vi "Teleop.vi"(10 "Match Info":T1={"Autonomous Elapsed Seconds"=0.0, "TeleOp Elapsed Seconds"=0.0, "Disabled Elapsed Seconds"=0.0, "Visited Autonomous"=FALSE, "Visited TeleOp"=FALSE, "Visited Disabled"=FALSE, "Autonomous Settings"={"Autonomous Style"=enum."Independent", "VI Refnum"=refnum}}, 11 "Call Context":T2) -> ()   [LabVIEW 2017]
doc: "This VI is called for each TeleOp packet received from the DS where the robot is not disabled. It is often used to read from the joysticks and update I/O or to update setpoints for timed control loops. It should complete and return within 20 milliseconds or it may miss DS packets."
uses:
  <vilib>/Rock Robotics/WPI/DriverStation/WPI_DriverStationDerivedRobotMode.ctl
  <vilib>/Rock Robotics/WPI/DriverStation/WPI_DriverStationMatch Info.ctl
  Phoenix-LabVIEW/Motor Controller/Controls/CTRE_Phoenix_MotorControl_ControlMode.ctl
  <vilib>/Rock Robotics/WPI/ThirdParty/Sensors/navX/_TypeDefs/FRIC_navX_DeviceNumbersTypeDef.ctl
  <vilib>/Rock Robotics/WPI/Utilities/WPI_GetSetVariantRefNum.vi
panel:
  in  "LiftSpeed":dbl=1.0 format="%#_13g"
  in  "LiftSetpoint":dbl=0.45 format="%#_13g"
  in  "Lift PID":bool
  in  "WristSetpoint":dbl format="%#_13g"
  in  "WristSpeed":dbl=1.0 format="%#_13g"
  in  "Wrist PID":bool
  out "RightOut":dbl
  out "LeftOut":dbl
  in  "K Constant":dbl=-1.0 format="%#_13g"
  in  "Deadband":dbl=0.05 format="%#_13g"
  in  "DriveSpeed":dbl=0.95 format="%#_13g"
  in  "IntakeSpeed":dbl=0.9
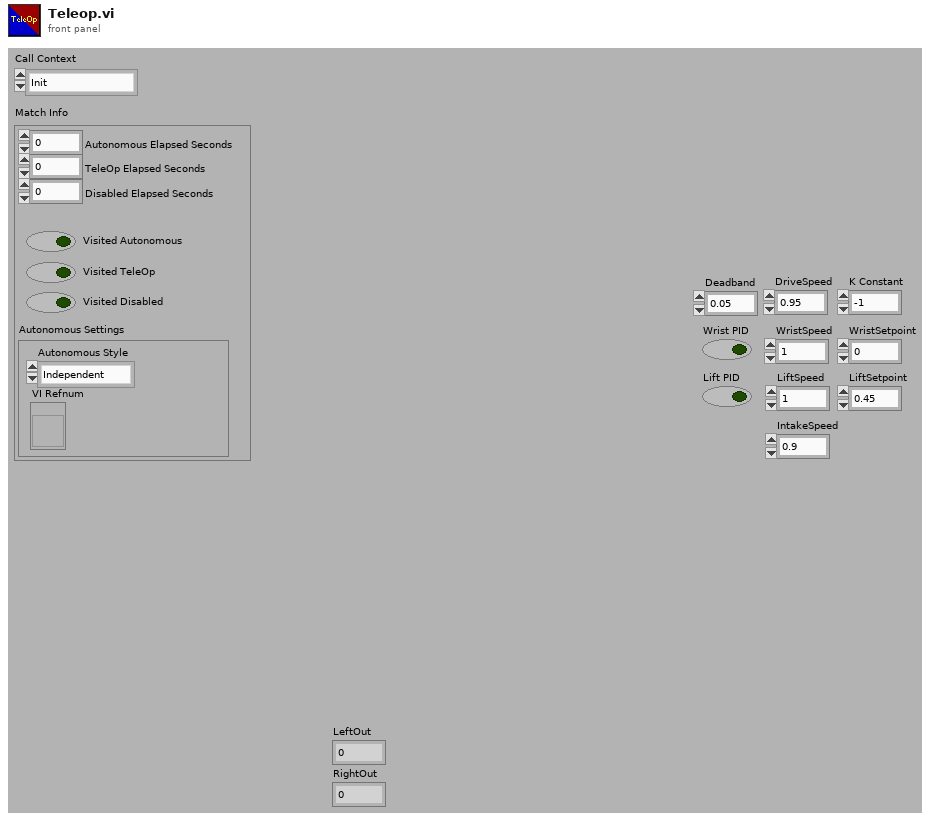
[diagram p1: front panel]
types:
  T1 = typedef "WPI_DriverStationMatch Info.ctl" = cluster{"Autonomous Elapsed Seconds":dbl, "TeleOp Elapsed Seconds":dbl, "Disabled Elapsed Seconds":dbl, "Visited Autonomous":bool, "Visited TeleOp":bool, "Visited Disabled":bool, "Autonomous Settings":cluster{"Autonomous Style":enum16{"Iterative", "Independent"}, "VI Refnum":refnum<vi>}}
  T2 = typedef "WPI_DriverStationDerivedRobotMode.ctl" = enum16{"Init", "Execute", "Stop"}
  T3 = typedef "CTRE_Phoenix_MotorControl_ControlMode.ctl" = u16
  T4 = typedef "WPI_JoystickDevRef.ctl" = cluster{"Device":T5}
  T5 = typedef "WPI_JoystickDeviceEnum.ctl" = enum16{"USB 0", "USB 1", "USB 2", "USB 3", "USB 4", "USB 5"}
  T6 = cluster{"Axes[0]":dbl, "Axes[1]":dbl, "Axes[2]":dbl, "Axes[3]":dbl, "Axes[4]":dbl, "Axes[5]":dbl, "Axes[6]":dbl, "Axes[7]":dbl, "Axes[8]":dbl}
  T7 = cluster{"Buttons[0]":bool, "Buttons[1]":bool, "Buttons[2]":bool, "Buttons[3]":bool, "Buttons[4]":bool, "Buttons[5]":bool, "Buttons[6]":bool, "Buttons[7]":bool, "Buttons[8]":bool}
  T8 = typedef "FRIC_navX_DeviceNumbersTypeDef.ctl" = enum16{"Dev0", "Dev1", "Dev2", "Dev3"}
  T9 = typedef "WPI_MotorControlDeviceRef.ctl" = cluster{"DeviceStatus":errorcluster, "Type":T10, "PWM":cluster{"PWM Channel":T11, "DeadBand":T12}, "CAN":cluster{"Device Number":u8, "SetOutput VI Ref":variant, "GetOutput VI Ref":variant, "Enable VI Ref":variant, "Disable VI Ref":variant, "Data":variant}, "Invert":bool, "DIO PWM":cluster{"PWM \"Enable\" Channel":T11, "DIOChannel":T13, "PWM Rate":dbl}}
  T10 = typedef "WPI_MotorControlType.ctl" = enum16{"PWM", "CAN", "DIO PWM"}
  T11 = typedef "FPGA_DIOPWMChannel.ctl" = enum8{"PWM 0", "PWM 1", "PWM 2", "PWM 3", "PWM 4", "PWM 5", "PWM 6", "PWM 7", "PWM 8", "PWM 9", "PWM MXP 0", "PWM MXP 1", "PWM MXP 2", "PWM MXP 3", "PWM MXP 4", "PWM MXP 5", "PWM MXP 6", "PWM MXP 7", "PWM MXP 8", "PWM MXP 9", "Invalid"}
  T12 = typedef "WPI_PWMDeadband.ctl" = cluster{"Name":string, "maxPositivePwm":i32, "minPositivePwm":i32, "centerPwm":i32, "maxNegativePwm":i32, "minNegativePwm":i32, "angularRange":u16}
  T13 = typedef "FPGA_DIOChannel.ctl" = enum8{"DIO 0", "DIO 1", "DIO 2", "DIO 3", "DIO 4", "DIO 5", "DIO 6", "DIO 7", "DIO 8", "DIO 9", "DIO MXP 0", "DIO MXP 1", "DIO MXP 2", "DIO MXP 3", "DIO MXP 4", "DIO MXP 5", "DIO MXP 6", "DIO MXP 7", "DIO MXP 8", "DIO MXP 9", "DIO MXP 10", "DIO MXP 11", "DIO MXP 12", "DIO MXP 13", "DIO MXP 14", "DIO MXP 15", "SPI Port CS1", "SPI Port CS2", "SPI Port CS3", "SPI Port MISO", "SPI Port MOSI", "Invalid"}
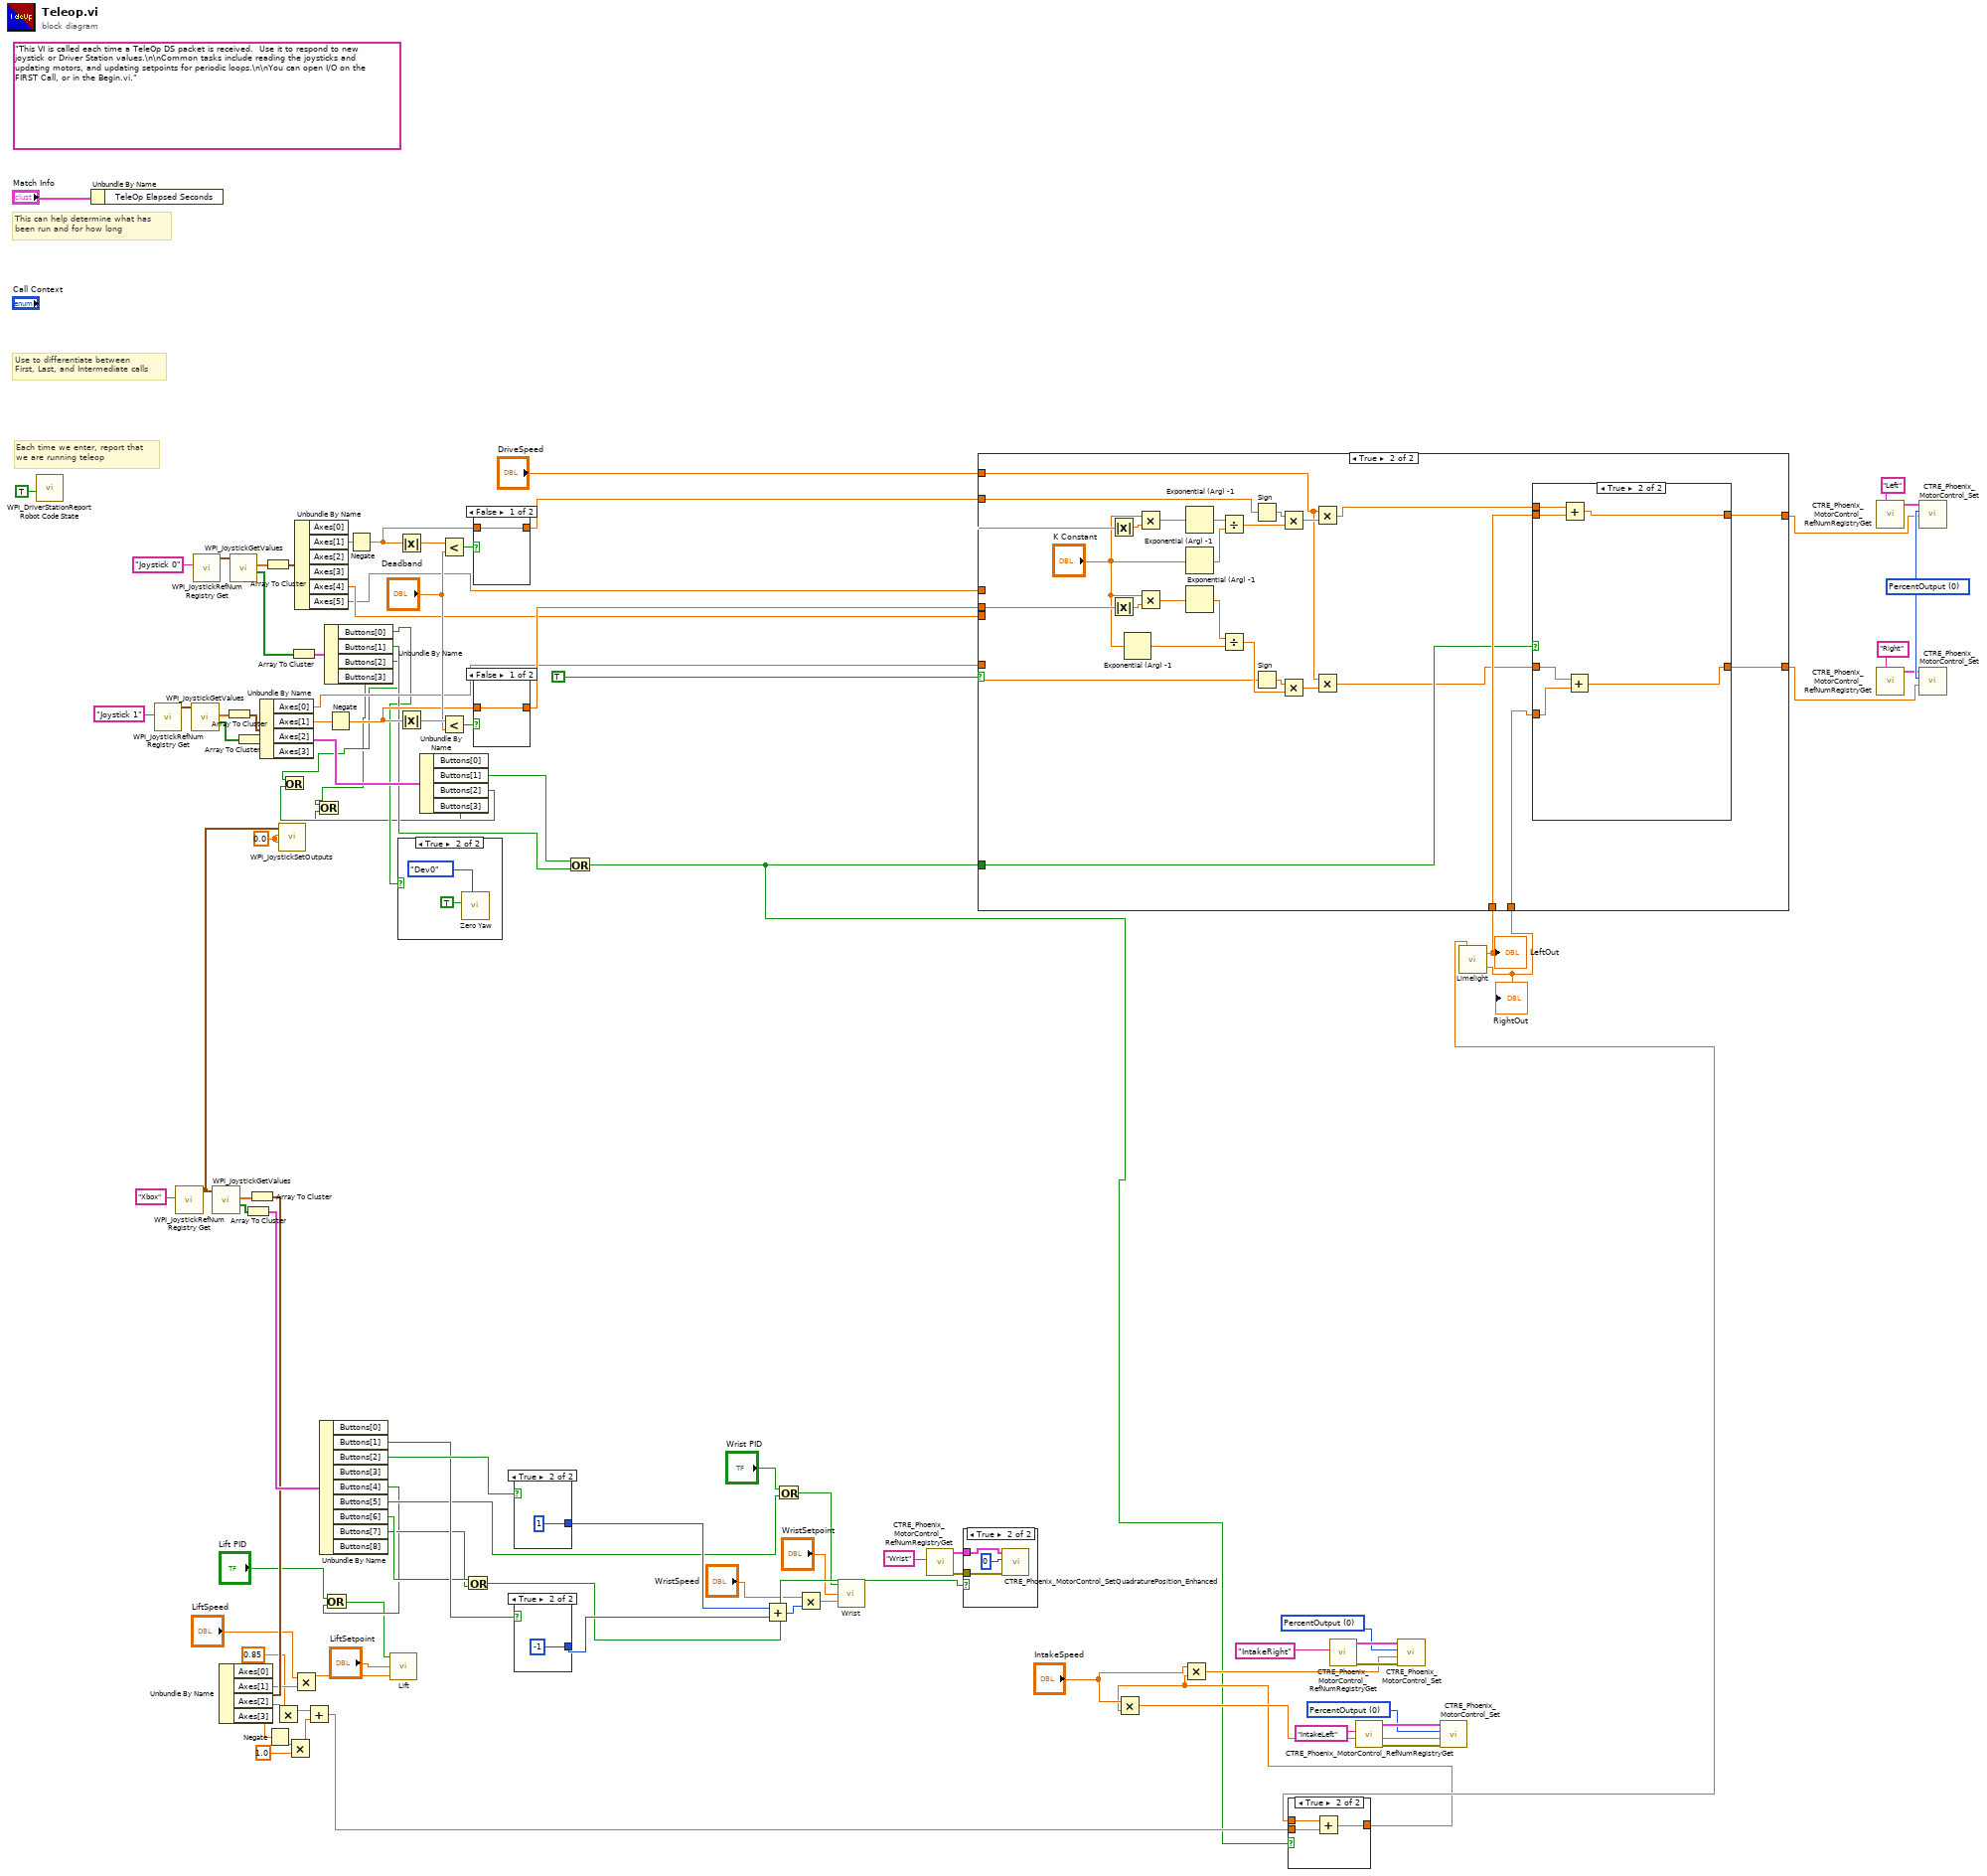
[diagram p0: block diagram]
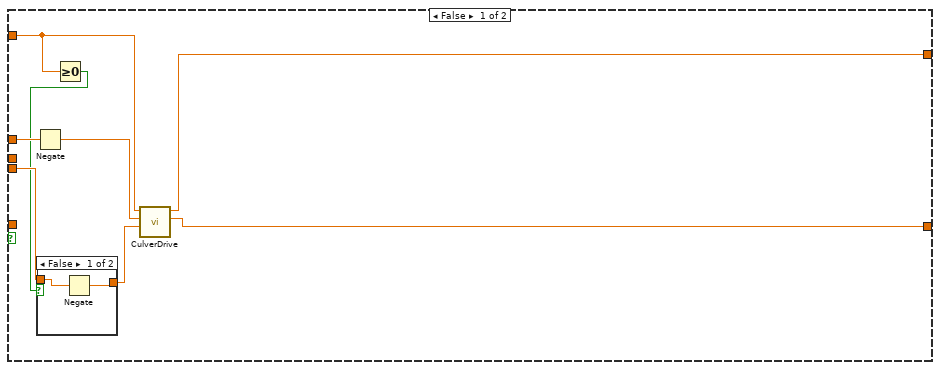
[diagram p5: hidden frame]
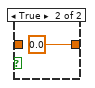
[diagram p8: hidden frame]
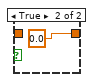
[diagram p9: hidden frame]
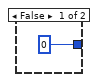
[diagram p10: hidden frame]
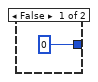
[diagram p11: hidden frame]
diagram:
  w48 = sgl 0.0 ("Left Rumble")
  w82 = T3 0 items=["PercentOutput"=0, "Position"=1, "Velocity"=2, "Current"=3, "Follower"=5, "MotionProfile"=6, "MotionMagic"=7, "MotionMagicArc"=8, "MotionProfileArc"=10, "Disabled"=15] ("Control Mode")
  w85 = T3 0 items=["PercentOutput"=0, "Position"=1, "Velocity"=2, "Current"=3, "Follower"=5, "MotionProfile"=6, "MotionMagic"=7, "MotionMagicArc"=8, "MotionProfileArc"=10, "Disabled"=15] ("Control Mode")
  w89 = T3 0 items=["PercentOutput"=0, "Position"=1, "Velocity"=2, "Current"=3, "Follower"=5, "MotionProfile"=6, "MotionMagic"=7, "MotionMagicArc"=8, "MotionProfileArc"=10, "Disabled"=15] ("Control Mode")
  (unwired) "This VI is called each time a TeleOp DS packet is received.  Use it to respond to new joystick or Driver Station values.\n\nCommon tasks include reading the joysticks and updating motors, and updating setpoints for periodic loops.\n\nYou can open I/O on the FIRST Call, or in the Begin.vi."
  # "Each time we enter, report that\nwe are running teleop"
  # "Use to differentiate between\nFirst, Last, and Intermediate calls"
  # "This can help determine what has\nbeen run and for how long"
  n1 = call <vilib>:"WPI_DriverStationReport Robot Code State.vi"("TeleOp"=TRUE ("Autonomous")) -> ()  [unwired: 10 in, 1 out]
  n2 = Unbundle By Name("Match Info") -> ()  [unwired: 1 out]
  n3 = call <vilib>:"WPI_JoystickRefNum Registry Get.vi"("refnum name"="Joystick 1") -> ("JoystickDevRef"=w52:T4)  [unwired: 1 in, 9 out]
  n4 = call <vilib>:"WPI_JoystickRefNum Registry Get.vi"("refnum name"="Xbox") -> ("JoystickDevRef"=w49:T4)  [unwired: 1 in, 9 out]
  n5 = call <vilib>:"WPI_JoystickGetValues.vi"("JoystickDevRef"=w52) -> ("Buttons"=w56:bool[], "Axes"=w76:dbl[])  [unwired: 6 in, 3 out]
  n6 = call <vilib>:"WPI_JoystickRefNum Registry Get.vi"("refnum name"="Joystick 0") -> ("JoystickDevRef"=w53:T4)  [unwired: 1 in, 9 out]
  n7 = call <vilib>:"WPI_JoystickGetValues.vi"("JoystickDevRef"=w49) -> ("Buttons"=w69:bool[], "Axes"=w70:dbl[])  [unwired: 6 in, 3 out]
  n8 = Array To Cluster(array=w76) -> (cluster=w75:T6)
  n9 = call <vilib>:"WPI_JoystickGetValues.vi"("JoystickDevRef"=w53) -> ("Buttons"=w80:bool[], "Axes"=w81:dbl[])  [unwired: 6 in, 3 out]
  n10 = Array To Cluster(array=w56) -> (cluster=w55:T7)
  n11 = Array To Cluster(array=w69) -> (cluster=w68:T7)
  n12 = Array To Cluster(array=w70) -> (cluster=w67:T6)
  n13 = Unbundle By Name(w67) -> ("Axes[1]"=w12:dbl, "Axes[2]"=w43:dbl, "Axes[3]"=w42:dbl)  [unwired: 1 out]
  n14 = Unbundle By Name(w75) -> ("Axes[0]"=w46:dbl, "Axes[1]"=w57:dbl)  [unwired: 2 out]
  n15 = Array To Cluster(array=w81) -> (cluster=w79:T6)
  n16 = Negate(x=w42) -> (-x=w4:dbl)
  n17 = Multiply(x=w43, y=0.85) -> (x*y=w2:dbl)
  n18 = call <vilib>:"WPI_JoystickSetOutputs.vi"("Right Rumble"=w48, "Left Rumble"=w48, "JoystickDevRef"=w49) -> ()  [unwired: 7 in, 2 out]
  n19 = Multiply(x=w4, y=1.0) -> (x*y=w5:dbl)
  n20 = Array To Cluster(array=w80) -> (cluster=w78:T7)
  n21 = Multiply(x="LiftSpeed", y=w12) -> (x*y=w7:dbl)
  n22 = Unbundle By Name(w79) -> ("Axes[1]"=w59:dbl, "Axes[4]"=w45:dbl, "Axes[5]"=w44:dbl)  [unwired: 3 out]
  n23 = Add(x=w2, y=w5) -> (x+y=w41:dbl)
  n24 = Unbundle By Name(w68) -> ("Buttons[1]"=w66:bool, "Buttons[2]"=w94:bool, "Buttons[4]"=w10:bool, "Buttons[5]"=w21:bool, "Buttons[6]"=w27:bool, "Buttons[7]"=w26:bool)  [unwired: 3 out]
  n25 = Or(x="Lift PID", y=w10) -> (x .or. y?=w9:bool)
  n26 = Unbundle By Name(w78) -> ("Buttons[0]"=w33:bool, "Buttons[1]"=w38:bool, "Buttons[2]"=w32:bool, "Buttons[3]"=w30:bool)
  n27 = Negate(x=w57) -> (-x=w50:dbl)
  n28 = Negate(x=w59) -> (-x=w51:dbl)
  n29 = call "Lift.vi"("LiftInput"=w7, "LiftSet"="LiftSetpoint", "LiftSweet"=w9) -> ()
  n30 = Absolute Value(x=w51) -> (abs(x)=w64:dbl)
  n31 = Absolute Value(x=w50) -> (abs(x)=w62:dbl)
  n32 = case shown="True" w33 {
    frame False {
    }
    frame True {
      n33 = call <vilib>:"Zero Yaw.vi"("Device Number"=FRIC_navX_DeviceNumbersTypeDef."Dev0", "Zero"=TRUE) -> ()  [unwired: 10 in]
    }
  }
  n34 = Unbundle By Name(w55) -> ("Buttons[1]"=w54:bool, "Buttons[2]"=w31:bool, "Buttons[3]"=w29:bool)  [unwired: 1 out]
  n35 = Or(x=w32, y=w31) -> ()  [unwired: 1 out]
  n36 = Or(x=w30, y=w29) -> ()  [unwired: 1 out]
  n37 = Less?(x=w64, y="Deadband") -> (x < y?=w65:bool)
  n38 = Less?(x=w62, y="Deadband") -> (x < y?=w63:bool)
  n39 = Or(x=w27, y=w26) -> (x .or. y?=w25:bool)
  n40 = case shown="False" w65 {
    tunnel: w51 -> [w102 _]
    tunnel: [w102 0.0] -> w61
    frame False {
    }
    frame True {
    }
  }
  n41 = case shown="False" w63 {
    tunnel: w50 -> [w104 _]
    tunnel: [w104 0.0] -> w60
    frame False {
    }
    frame True {
    }
  }
  n42 = case shown="True" w94 {
    tunnel: [0 1] -> w92
    frame False {
    }
    frame True {
    }
  }
  n43 = case shown="True" w66 {
    tunnel: [0 -1] -> w95
    frame False {
    }
    frame True {
    }
  }
  n44 = Or(x=w54, y=w38) -> (x .or. y?=w34:bool)
  n45 = Add(x=w92, y=w95) -> (x+y=w19:i32)
  n46 = Or(x="Wrist PID", y=w21) -> (x .or. y?=w20:bool)
  n47 = Multiply(x="WristSpeed", y=w19) -> (x*y=w18:dbl)
  n48 = call "Wrist.vi"("WristInput"=w18, "WristSetpoint"="WristSetpoint", "WristSweet"=w20) -> ()
  n49 = call "CTRE_Phoenix_MotorControl_RefNumRegistryGet.vi"("refnum name"="Wrist") -> ("error out"=w13:errorcluster, "PhoenixMotorControlDevRef"=w14:T9)  [unwired: 9 in]
  n50 = case shown="True" w25 {
    tunnel: w14 -> [_ w111]
    tunnel: w13 -> [_ w110]
    frame False {
    }
    frame True {
      n51 = call <vilib>:"CTRE_Phoenix_MotorControl_SetQuadraturePosition_Enhanced.vi"("error in (no error)"=w110, "New Position"=0, "PhoenixMotorControlDevRef"=w111) -> ()  [unwired: 7 in, 2 out]
    }
  }
  n52 = call "CTRE_Phoenix_MotorControl_RefNumRegistryGet.vi"("refnum name"="IntakeRight") -> ("error out"=w90:errorcluster, "PhoenixMotorControlDevRef"=w91:T9)  [unwired: 9 in]
  n53 = call "CTRE_Phoenix_MotorControl_RefNumRegistryGet.vi"("refnum name"="IntakeLeft") -> ("error out"=w86:errorcluster, "PhoenixMotorControlDevRef"=w87:T9)  [unwired: 9 in]
  n54 = call "Limelight.vi"() -> ("RightOut"=w39:dbl, "LeftOut"=w40:dbl, "IntakeOut"=w36:dbl)  [unwired: 1 in]
  "LeftOut" <- w40
  "RightOut" <- w39
  n55 = case shown="True" TRUE {
    tunnel: w61 -> [w116 w136]
    tunnel: w60 -> [_ w135]
    tunnel: [w119 w128] -> w23
    tunnel: [w120 w130] -> w24
    tunnel: w46 -> [_ _]
    tunnel: w45 -> [w115 _]
    tunnel: w44 -> [w118 _]
    tunnel: w40 -> [_ w131]
    tunnel: w39 -> [_ w129]
    tunnel: w34 -> [_ w127]
    tunnel: "DriveSpeed" -> [_ w124]
    frame False {
      n56 = Negate(x=w118) -> (-x=w117:dbl)
      n57 = Greater Or Equal To 0?(x=w116) -> (x >= 0?=w114:bool)
      n58 = case shown="False" w114 {
        tunnel: w115 -> [w121 w123]
        tunnel: [w122 w123] -> w113
        frame False {
          n59 = Negate(x=w121) -> (-x=w122:dbl)
        }
        frame True {
        }
      }
      n60 = call "CulverDrive.vi"("Wheel.X"=w113, "Wheel.Y"=w117, "Throttle"=w116) -> ("Right Side"=w119:dbl, "Left Side"=w120:dbl)  [unwired: 5 in, 2 out]
    }
    frame True {
      n61 = Absolute Value(x=w136) -> (abs(x)=w142:dbl)
      n62 = Absolute Value(x=w135) -> (abs(x)=w141:dbl)
      n63 = Exponential (Arg) -1(1:"K Constant") -> (0:w145:dbl)
      n64 = Multiply(x="K Constant", y=w142) -> (x*y=w146:dbl)
      n65 = Multiply(x="K Constant", y=w141) -> (x*y=w143:dbl)
      n66 = Exponential (Arg) -1(1:w146) -> (0:w147:dbl)
      n67 = Exponential (Arg) -1(1:"K Constant") -> (0:w148:dbl)
      n68 = Exponential (Arg) -1(1:w143) -> (0:w144:dbl)
      n69 = Divide(x=w147, y=w148) -> (x/y=w139:dbl)
      n70 = Divide(x=w144, y=w145) -> (x/y=w137:dbl)
      n71 = Sign(1:w136) -> (0:w140:dbl)
      n72 = Sign(1:w135) -> (0:w138:dbl)
      n73 = Multiply(x=w140, y=w139) -> (x*y=w133:dbl)
      n74 = Multiply(x=w138, y=w137) -> (x*y=w132:dbl)
      n75 = Multiply(x=w124, y=w133) -> (x*y=w126:dbl)
      n76 = Multiply(x=w124, y=w132) -> (x*y=w125:dbl)
      n77 = case shown="True" w127 {
        tunnel: w131 -> [_ w154]
        tunnel: [w150 w156] -> w130
        tunnel: w129 -> [_ w151]
        tunnel: [w149 w153] -> w128
        tunnel: w126 -> [w150 w155]
        tunnel: w125 -> [w149 w152]
        frame False {
        }
        frame True {
          n78 = Add(x=w155, y=w154) -> (x+y=w156:dbl)
          n79 = Add(x=w152, y=w151) -> (x+y=w153:dbl)
        }
      }
    }
  }
  n80 = case shown="True" w34 {
    tunnel: w36 -> [_ w160]
    tunnel: [w157 w159] -> w35
    tunnel: w41 -> [w157 w158]
    frame False {
    }
    frame True {
      n81 = Add(x=w160, y=w158) -> (x+y=w159:dbl)
    }
  }
  n82 = Multiply(x="IntakeSpeed", y=w35) -> (x*y=w84:dbl)
  n83 = Multiply(x="IntakeSpeed", y=w35) -> (x*y=w72:dbl)
  n84 = call "CTRE_Phoenix_MotorControl_Set.vi"("error in (no error)"=w90, "Output"=w72, "Control Mode"=w89, "PhoenixMotorControlDevRef"=w91) -> ()  [unwired: 6 in, 2 out]
  n85 = call "CTRE_Phoenix_MotorControl_Set.vi"("error in (no error)"=w86, "Output"=w84, "Control Mode"=w85, "PhoenixMotorControlDevRef"=w87) -> ()  [unwired: 6 in, 2 out]
  n86 = call "CTRE_Phoenix_MotorControl_RefNumRegistryGet.vi"("refnum name"="Left") -> ("PhoenixMotorControlDevRef"=w73:T9)  [unwired: 9 in, 1 out]
  n87 = call "CTRE_Phoenix_MotorControl_RefNumRegistryGet.vi"("refnum name"="Right") -> ("PhoenixMotorControlDevRef"=w74:T9)  [unwired: 9 in, 1 out]
  n88 = call "CTRE_Phoenix_MotorControl_Set.vi"("Output"=w24, "Control Mode"=w82, "PhoenixMotorControlDevRef"=w73) -> ()  [unwired: 7 in, 2 out]
  n89 = call "CTRE_Phoenix_MotorControl_Set.vi"("Output"=w23, "Control Mode"=w82, "PhoenixMotorControlDevRef"=w74) -> ()  [unwired: 7 in, 2 out]
